vi "Tosca-Display Adaptation Progress.vi"(0 "Track":T5, 5 "Track def":T1, 7 "Controls":T4, 11 "which":i32) -> (8 "Controls thru":T4)   [LabVIEW 2020]
uses:
  Typedefs/Tosca-Control Refs.ctl
  FSM Graph VIs/LV Source/FSM Editor/FSM Editor.xctl
  Typedefs/Tosca-Adaptation Track State.ctl
  Typedefs/Tosca-Adaptation History Element.ctl
  Typedefs/Tosca-Adaptive Track.ctl
  Typedefs/Tosca-Simple Variable.ctl
  Adaptation VIs/Tosca-Adapt Threshold Metric.ctl
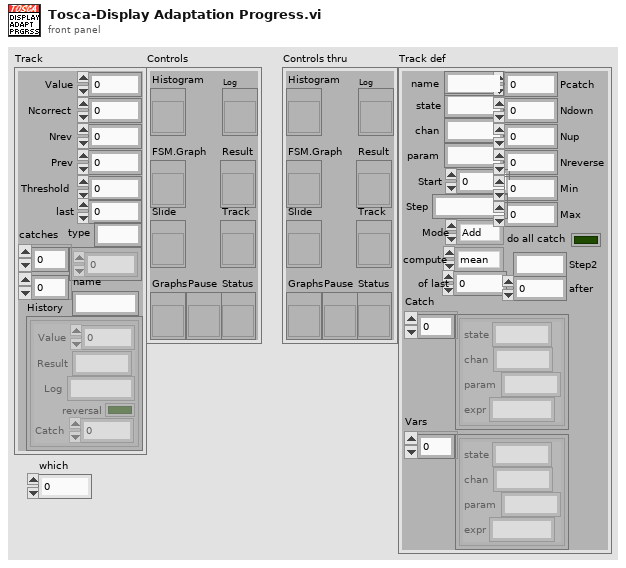
[diagram p1: front panel]
types:
  T1 = typedef "Tosca-Adaptive Track.ctl" = cluster{"state":string, "chan":string, "param":string, "Start":dbl, "Step":string, "Mode":enum16{"Add", "Multiply"}, "Pcatch":dbl, "Ndown":i32, "Nup":i32, "Nreverse":i32, "Min":dbl, "Max":dbl, "Catch":T2[], "do all catch":bool, "name":string, "Vars":T2[], "compute":T3, "of last":i32, "Step2":string, "after":i32}
  T2 = typedef "Tosca-Simple Variable.ctl" = cluster{"state":string, "chan":string, "param":string, "expr":string}
  T3 = typedef "Tosca-Adapt Threshold Metric.ctl" = enum16{"mean", "median"}
  T4 = typedef "Tosca-Control Refs.ctl" = cluster{"FSM.Graph":refnum<vi>, "Slide":refnum<vi>, "Result":refnum<vi>, "Histogram":refnum<vi>, "Graphs":refnum<vi>, "Track":refnum<vi>, "Log":refnum<vi>, "Status":refnum<vi>, "Pause":refnum<vi>}
  T5 = typedef "Tosca-Adaptation Track State.ctl" = cluster{"Value":dbl, "Ncorrect":i32, "Nrev":i32, "Prev":dbl, "History":T6[], "Threshold":dbl, "last":i32, "type":string, "catches":dbl[][], "name":string}
  T6 = typedef "Tosca-Adaptation History Element.ctl" = cluster{"Value":dbl, "Result":string, "Log":string, "reversal":bool, "Catch":dbl}
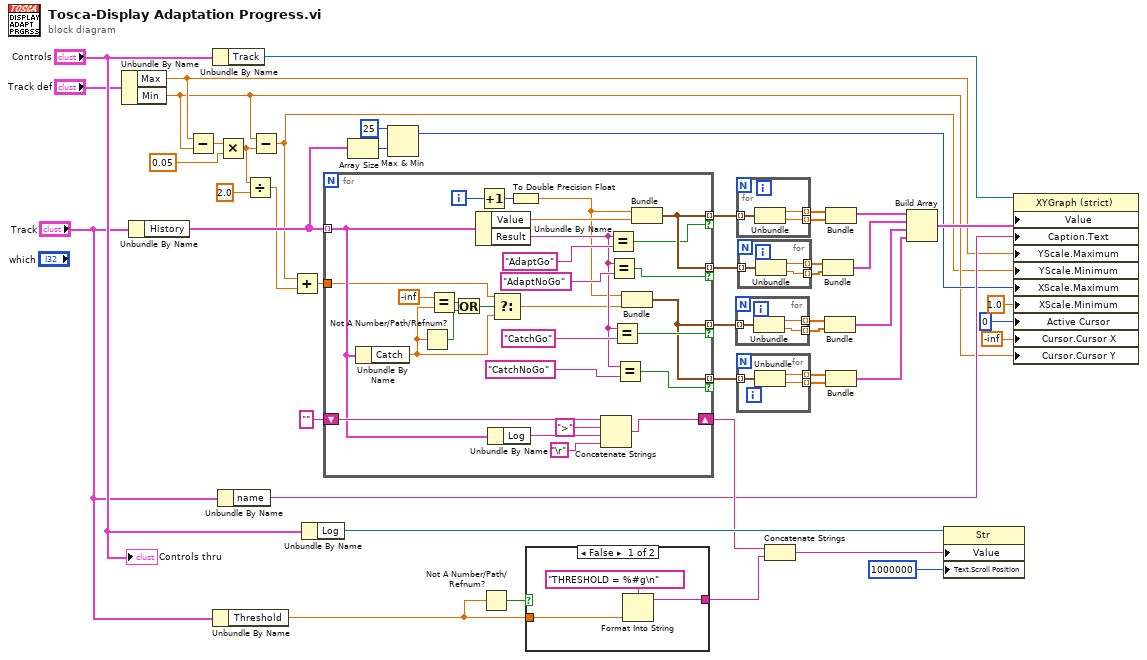
[diagram p0: block diagram]
diagram:
  n1 = Unbundle By Name("Track def") -> ("Max"=w11:dbl, "Min"=w6:dbl)
  n2 = Unbundle By Name("Track") -> ("History"=w15:T6[])
  n3 = Subtract(x=w11, y=w6) -> (x-y=w10:dbl)
  n4 = Unbundle By Name("Controls") -> ("Track"=w45:refnum<vi>)
  n5 = Unbundle By Name("Track") -> ("Threshold"=w25:dbl)
  n6 = Multiply(x=w10, y=0.05) -> (x*y=w5:dbl)
  n7 = Unbundle By Name("Track") -> ("name"=w22:string)
  n8 = Divide(x=w5, y=2.0) -> (x/y=w2:dbl)
  n9 = Subtract(x=w6, y=w5) -> (x-y=w1:dbl)
  n10 = Add(x=w1, y=w2) -> (x+y=w3:dbl)
  n11 = Unbundle By Name("Controls") -> ("Log"=w43:refnum<vi>)
  n12 = for {
    tunnel: w15 -> [w61] mode=indexing
    tunnel: [w59] -> w41 mode=indexing if=w58
    shift-right: [w64] -> w42
    shift-left: "" -> [w68]
    tunnel: [w54] -> w36 mode=indexing if=w63
    tunnel: [w54] -> w33 mode=indexing if=w62
    tunnel: [w59] -> w21 mode=indexing if=w57
    tunnel: w3 -> [w52]
    i -> [w74]
    n13 = Unbundle By Name(w61) -> ("Catch"=w50:dbl)
    n14 = Not A Number/Path/Refnum?(number/path/refnum=w50) -> (NaN/Path/Refnum?=w47:bool)
    n15 = Equal?(x=-inf, y=w50) -> (x = y?=w48:bool)
    n16 = Or(x=w48, y=w47) -> (x .or. y?=w49:bool)
    n17 = Unbundle By Name(w61) -> ("Value"=w56:dbl, "Result"=w70:string)
    n18 = Increment(x=w74) -> (x+1=w60:i32)
    n19 = Unbundle By Name(w61) -> ("Log"=w67:string)
    n20 = Select(t=w52, s=w49, f=w50) -> (s? t:f=w53:dbl)
    n21 = To Double Precision Float(number=w60) -> (double precision float=w55:dbl)
    n22 = Concatenate Strings(w68, ">" ("string"), w67, "\r") -> (w64:string)
    n23 = Equal?(x=w70, y="AdaptGo") -> (x = y?=w58:bool)
    n24 = Equal?(x=w70, y="AdaptNoGo") -> (x = y?=w57:bool)
    n25 = Equal?(x=w70, y="CatchGo") -> (x = y?=w63:bool)
    n26 = Equal?(x=w70, y="CatchNoGo") -> (x = y?=w62:bool)
    n27 = Bundle(w55, "Catch"=w53) -> (w54:cluster{dbl, "Catch":dbl})  [unwired: 1 in]
    n28 = Bundle(w55, "Value"=w56) -> (w59:cluster{dbl, "Value":dbl})  [unwired: 1 in]
  }
  n29 = Array Size(array=w15) -> (size(s)=w14:i32)
  n30 = Max & Min(x=25, y=w14) -> (max(x,y)=w12:i32)  [unwired: 1 out]
  n31 = Not A Number/Path/Refnum?(number/path/refnum=w25) -> (NaN/Path/Refnum?=w26:bool)
  n32 = case shown="False" w26 {
    tunnel: w25 -> [w76 _]
    tunnel: [w77 _] -> w24
    frame False {
      n33 = Format Into String(format string="THRESHOLD = %#g\n", w76) -> (resulting string=w77:string)  [unwired: 2 in, 1 out]
    }
    frame True {
    }
  }
  n34 = for {
    tunnel: w36 -> [w80] mode=indexing
    tunnel: [w79] -> w38 mode=indexing
    tunnel: [w78] -> w37 mode=indexing
    n35 = Unbundle(w80) -> (w79:dbl, "Catch"=w78:dbl)
  }
  n36 = for {
    tunnel: w41 -> [w83] mode=indexing
    tunnel: [w82] -> w40 mode=indexing
    tunnel: [w81] -> w39 mode=indexing
    n37 = Unbundle(w83) -> (w82:dbl, "Value"=w81:dbl)
  }
  n38 = for {
    tunnel: w33 -> [w86] mode=indexing
    tunnel: [w85] -> w35 mode=indexing
    tunnel: [w84] -> w34 mode=indexing
    n39 = Unbundle(w86) -> (w85:dbl, "Catch"=w84:dbl)
  }
  n40 = for {
    tunnel: w21 -> [w89] mode=indexing
    tunnel: [w88] -> w20 mode=indexing
    tunnel: [w87] -> w19 mode=indexing
    n41 = Unbundle(w89) -> (w88:dbl, "Value"=w87:dbl)
  }
  n42 = Concatenate Strings(w42, w24) -> (w27:string)
  n43 = Bundle(w20, w19) -> (w18:cluster{dbl[], dbl[]})  [unwired: 1 in]
  n44 = Bundle(w38, w37) -> (w31:cluster{dbl[], dbl[]})  [unwired: 1 in]
  n45 = Bundle(w40, w39) -> (w32:cluster{dbl[], dbl[]})  [unwired: 1 in]
  n46 = Bundle(w35, w34) -> (w30:cluster{dbl[], dbl[]})  [unwired: 1 in]
  n47 = Build Array(w32, w18, w31, w30) -> (w29:cluster{dbl[], dbl[]}[])
  n48 = property class="Str"(reference=w43, "Value"=w27, "Text.Scroll Position"=u32 1000000) -> ()  [unwired: 1 in, 2 out]
  n49 = property class="XYGraph (strict)"(reference=w45, "Value"=w29, "Caption.Text"=w22, "YScale.Maximum"=w11, "YScale.Minimum"=w1, "XScale.Maximum"=w12, "XScale.Minimum"=1.0 ("X Scale.Range:Minimum"), "Active Cursor"=u32 0, "Cursor.Cursor X"=-inf, "Cursor.Cursor Y"=w6) -> ()  [unwired: 1 in, 2 out]
  "Controls thru" <- "Controls"
